vi "余额查询.vi"() -> (0 "出账总额":string, 2 "进账总额":string)   [LabVIEW 2010]
panel:
  in  "error in (no error) 2":errorcluster caption="错误输入（无错误）"
  in  "error in (no error)":errorcluster caption="错误输入（无错误）"
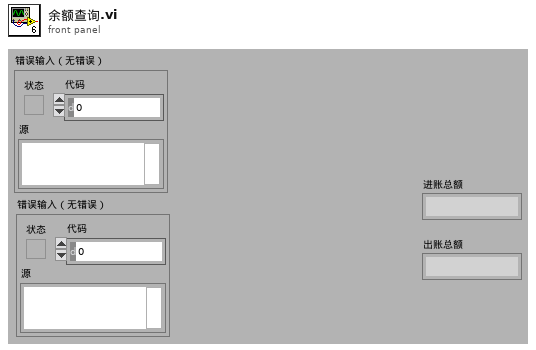
[diagram p1: front panel]
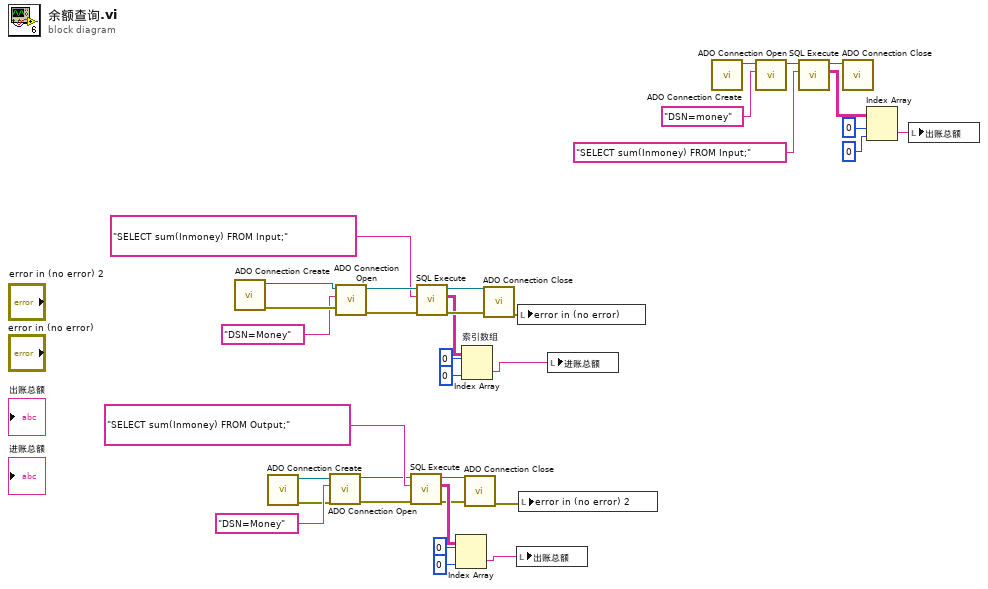
[diagram p0: block diagram]
diagram:
  n1 = call "ADO Connection Create.vi"() -> ("error out"=w35:errorcluster, "ADODB._Connection Out"=w10:refnum<k7>)  [unwired: 10 in]
  n2 = call "ADO Connection Create.vi"() -> ("error out"=w13:errorcluster, "ADODB._Connection Out"=w14:refnum<k7>)  [unwired: 10 in]
  n3 = call "ADO Connection Open.vi"("error in (no error)"=w13, "ConnectionString"="DSN=Money", "ADODB._Connection In"=w14) -> ("error out"=w16:errorcluster, "ADODB._Connection Out"=w15:refnum<k7>)  [unwired: 7 in]
  n4 = call "ADO Connection Open.vi"("error in (no error)"=w35, "ConnectionString"="DSN=Money", "ADODB._Connection In"=w10) -> ("error out"=w33:errorcluster, "ADODB._Connection Out"=w34:refnum<k7>)  [unwired: 7 in]
  n5 = call "SQL Execute.vi"("error in (no error)"=w16, "Command Text"="SELECT sum(Inmoney) FROM Output;", "ADODB._Connection In"=w15) -> ("error out"=w18:errorcluster, "Data"=w23:string[][], "ADODB._Connection Out"=w17:refnum<k7>)  [unwired: 5 in, 1 out]
  n6 = call "SQL Execute.vi"("error in (no error)"=w33, "Command Text"="SELECT sum(Inmoney) FROM Input;", "ADODB._Connection In"=w34) -> ("error out"=w31:errorcluster, "Data"=w25:string[][], "ADODB._Connection Out"=w32:refnum<k7>)  [unwired: 5 in, 1 out]
  n7 = Index Array(array=w23, index (row)=0 ("禁用的索引 (行)"), index (col)=0 ("禁用的索引 (列)")) -> (element=w12:string)
  n8 = Index Array "索引数组"(array=w25, index (row)=0 ("禁用的索引 (行)"), index (col)=0 ("禁用的索引 (列)")) -> (element=w27:string)
  n9 = call "ADO Connection Close.vi"("error in (no error)"=w18, "ADODB._Connection In"=w17) -> ("error out"=w11:errorcluster)  [unwired: 8 in, 1 out]
  n10 = call "ADO Connection Close.vi"("error in (no error)"=w31, "ADODB._Connection In"=w32) -> ("error out"=w24:errorcluster)  [unwired: 8 in, 1 out]
  n11 = local write "出账总额"(w12) -> ()
  n12 = local write "error in (no error)"(w24) -> ()
  n13 = local write "error in (no error) 2"(w11) -> ()
  n14 = local write "进账总额"(w27) -> ()
  n15 = call "ADO Connection Create.vi"() -> ("ADODB._Connection Out"=w9:refnum<k7>)  [unwired: 10 in, 1 out]
  n16 = call "ADO Connection Open.vi"("ConnectionString"="DSN=money", "ADODB._Connection In"=w9) -> ("ADODB._Connection Out"=w7:refnum<k7>)  [unwired: 8 in, 1 out]
  n17 = call "SQL Execute.vi"("Command Text"="SELECT sum(Inmoney) FROM Input;", "ADODB._Connection In"=w7) -> ("Data"=w5:string[][], "ADODB._Connection Out"=w1:refnum<k7>)  [unwired: 6 in, 2 out]
  n18 = call "ADO Connection Close.vi"("ADODB._Connection In"=w1) -> ()  [unwired: 9 in, 2 out]
  n19 = Index Array(array=w5, index (row)=0 ("索引 (行)"), index (col)=0 ("禁用的索引 (列)")) -> (element=w2:string)
  n20 = local write "出账总额"(w2) -> ()
